vi "Merge Cells.vi"(8 "error in":errorcluster, 10 "Cell Parameters":T1={"Cell Range"="", "Horizontal Alignment"=enum."xlcenter", "Vertical Alignment"=enum."xlcentet"}, 11 "_Worksheet":refnum<k7>) -> (0 "error out":errorcluster, 3 "_Worksheet":refnum<k7>)   [LabVIEW 2017]
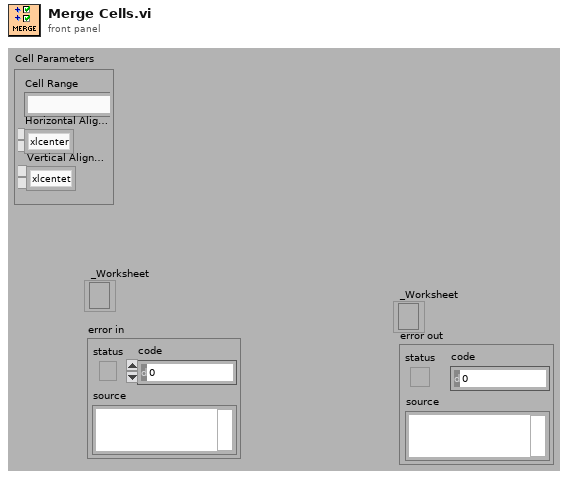
[diagram p1: front panel]
types:
  T1 = cluster{"Cell Range":string, "Horizontal Alignment":enum16{"xlnone", "xlgeneral", "xlleft", "xlcenter", "xlright"}, "Vertical Alignment":enum16{"xlnone", "xltop", "xlcentet", "xlbottom"}}
  T2 = enum16{"xlnone", "xlgeneral", "xlleft", "xlcenter", "xlright"}
  T3 = enum16{"xlnone", "xltop", "xlcentet", "xlbottom"}
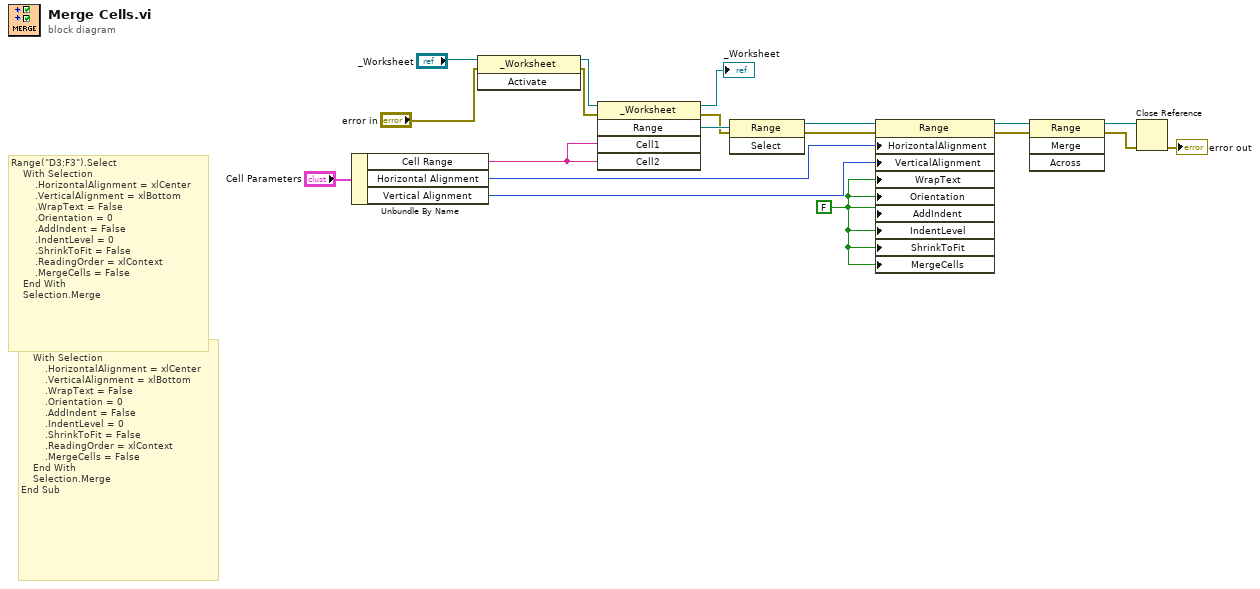
[diagram p0: block diagram]
diagram:
  w15 = FALSE
  # "Range(\"A3:F3\").Select\n    With Selection\n        .HorizontalAlignment = xlCenter\n        .VerticalAlignment = xlBottom\n        .WrapText = False\n        .Orientation = 0\n        .AddIndent = False\n        .IndentLevel = 0\n        .ShrinkToFit = False\n        .ReadingOrder = xlContext\n        .MergeCells = False\n    End With\n    Selection.Merge\nEnd Sub"
  # "Range(\"D3:F3\").Select\n    With Selection\n        .HorizontalAlignment = xlCenter\n        .VerticalAlignment = xlBottom\n        .WrapText = False\n        .Orientation = 0\n        .AddIndent = False\n        .IndentLevel = 0\n        .ShrinkToFit = False\n        .ReadingOrder = xlContext\n        .MergeCells = False\n    End With\n    Selection.Merge"
  n1 = Unbundle By Name("Cell Parameters") -> ("Cell Range"=w5:string, "Horizontal Alignment"=w7:T2, "Vertical Alignment"=w6:T3)
  n2 = invoke class="_Worksheet" method="Activate"(reference="_Worksheet", error in="error in") -> (reference out=w3:refnum<k7>, error out=w1:errorcluster)  [unwired: 1 in, 1 out]
  n3 = invoke class="_Worksheet" method="Range"(reference=w3, error in=w1, "Cell1"=w5, "Cell2"=w5) -> (reference out=→"_Worksheet":refnum<k7>, error out=w18:errorcluster, "Range"=w19:refnum<k7>)  [unwired: 1 in, 2 out]
  n4 = invoke class="Range" method="Select"(reference=w19, error in=w18) -> (reference out=w17:refnum<k7>, error out=w16:errorcluster)  [unwired: 1 in, 1 out]
  n5 = property class="Range"(reference=w17, error in=w16, "HorizontalAlignment"=w7, "VerticalAlignment"=w6, "WrapText"=w15, "Orientation"=w15, "AddIndent"=w15, "IndentLevel"=w15, "ShrinkToFit"=w15, "MergeCells"=w15) -> (reference out=w14:refnum<k7>, error out=w13:errorcluster)
  n6 = invoke class="Range" method="Merge"(reference=w14, error in=w13) -> (reference out=w12:refnum<k7>, error out=w11:errorcluster)  [unwired: 2 in, 2 out]
  n7 = Close Reference(reference=w12, error in (no error)=w11) -> (error out=→"error out":errorcluster)
